vi "State Flow Test Timer.vi"() -> ()   [LabVIEW 2013]
panel:
  out "Boolean":bool
  out "Elapsed Time (s)":dbl
  in  "Button":bool
  out "State 3":bool
  out "State 2":bool
  out "State 1":bool
  out "State 0":bool
  out "State":dbl
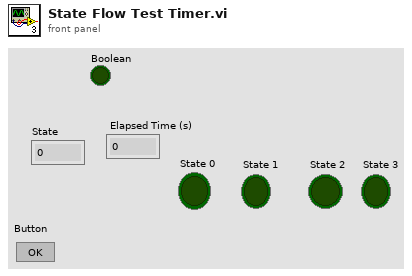
[diagram p1: front panel]
types:
  T1 = enum16{"Release Lock", "Pullback On", "Lock On", "Pullback Off"}
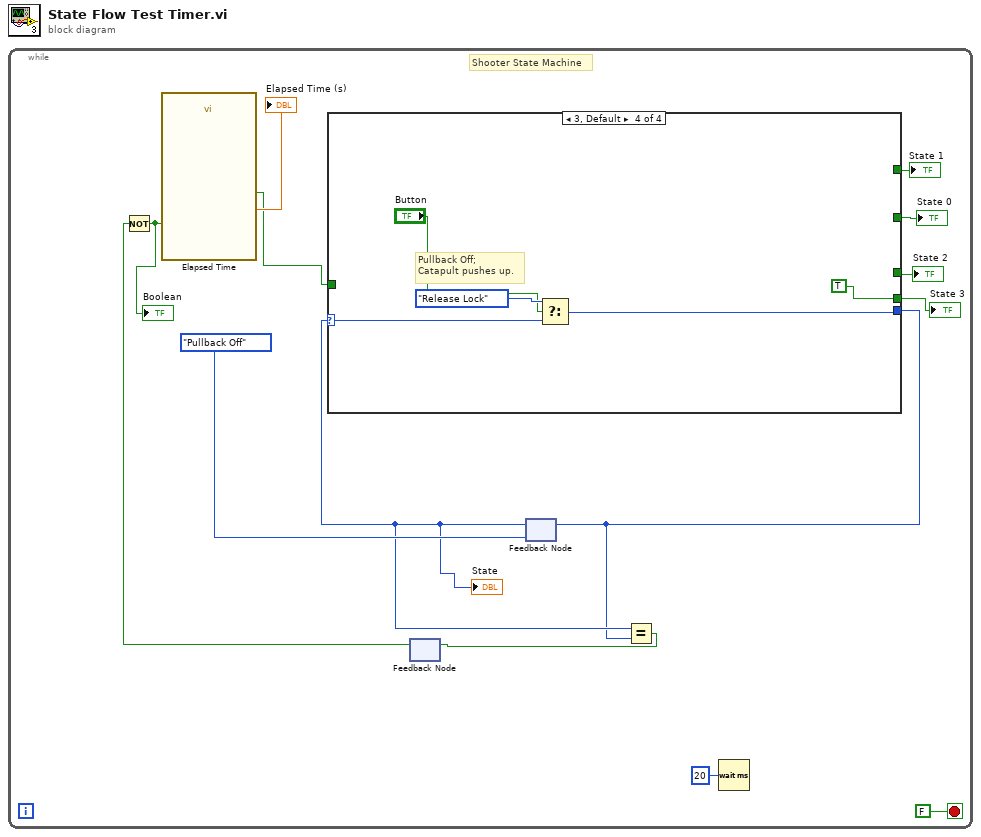
[diagram p0: block diagram]
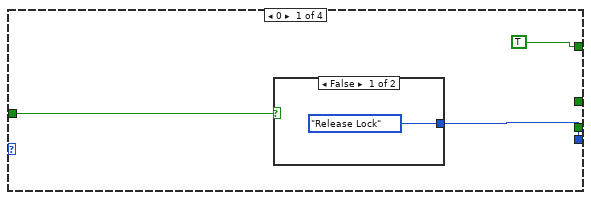
[diagram p2: hidden frame]
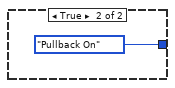
[diagram p3: hidden frame]
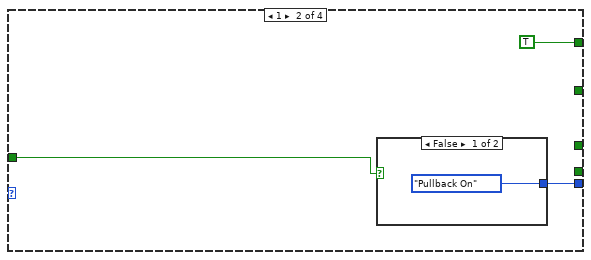
[diagram p4: hidden frame]
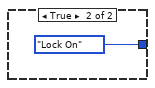
[diagram p5: hidden frame]
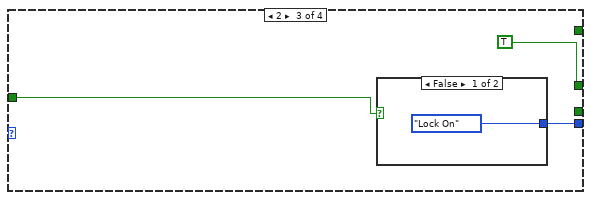
[diagram p6: hidden frame]
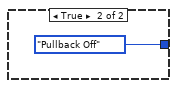
[diagram p7: hidden frame]
diagram:
  n1 = while {
    stop <- FALSE stop-if-true
    # "Shooter State Machine"
    n2 = feedback #1() -> (w3:bool)  [unwired: 1 in]
    n3 = Not(x=w3) -> (.not. x?=w1:bool)
    "Boolean" <- w1
    n4 = call "Elapsed Time"("Reset"=w1) -> ("Elapsed Time (s)"=→"Elapsed Time (s)":dbl, "Time has Elapsed"=w2:bool)  [unwired: 11 in, 6 out]
    n5 = feedback #2(T1."Pullback Off") -> (w7:u32)
    "State" <- w7
    n6 = case shown="3, Default" w7 {
      selector: w7 -> [_ _ _ w32]
      tunnel: [w17 w22 w27 w34] -> w6
      tunnel: [TRUE ("State 0") _ _ _] -> w13
      tunnel: [_ TRUE _ _] -> w12
      tunnel: [_ _ TRUE _] -> w11
      tunnel: [_ _ _ TRUE] -> w10
      tunnel: w2 -> [w15 w20 w25 _]
      frame 0 {
        n7 = case shown="False" w15 {
          tunnel: [T1."Release Lock" T1."Pullback On"] -> w17
          frame False {
          }
          frame True {
          }
        }
      }
      frame 1 {
        n8 = case shown="False" w20 {
          tunnel: [T1."Pullback On" T1."Lock On"] -> w22
          frame False {
          }
          frame True {
          }
        }
      }
      frame 2 {
        n9 = case shown="False" w25 {
          tunnel: [T1."Lock On" T1."Pullback Off"] -> w27
          frame False {
          }
          frame True {
          }
        }
      }
      frame 3, Default {
        # "Pullback Off;\nCatapult pushes up."
        n10 = Select(t=T1."Release Lock", s="Button", f=w32) -> (s? t:f=w34:u32)
      }
    }
    "State 0" <- w13
    "State 2" <- w11
    "State 1" <- w12
    "State 3" <- w10
    n11 = feedback-in #2(w6) -> ()
    n12 = Equal?(x=w7, y=w6) -> (x = y?=w4:bool)
    n13 = feedback-in #1(w4) -> ()
    n14 = Wait (ms)(milliseconds to wait=u32 20) -> ()  [unwired: 1 out]
  }
